vi "Add Or Update Attribute.vi"(8 "error in (no error)":errorcluster, 10 "Atrribute":refnum<class "Attribute.lvclass">, 11 "Object in":refnum<class "Object.lvclass">) -> (0 "error out":errorcluster, 3 "Object out":refnum<class "Object.lvclass">)   [LabVIEW 2019, in "HierDAL Library.lvlib" / "Models.lvlib" / "Object.lvclass"]
uses:
  Object.lvclass
  Attribute Class/Attribute.lvclass
  Object.lvclass/Object.ctl
  Attribute Class/Attribute.lvclass/Attribute.ctl
  d909fb08-bf4f-481c-9526-163c37e898ac.vi
  Attribute Class/Get Key.vi
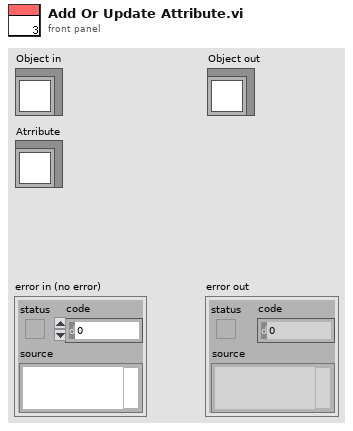
[diagram p1: front panel]
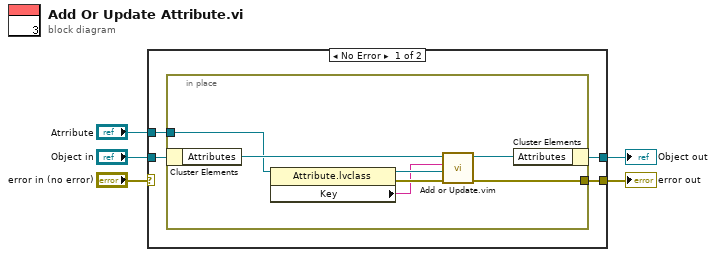
[diagram p0: block diagram]
diagram:
  n1 = case shown="No Error" "error in (no error)" {
    selector: "error in (no error)" -> [_ w18]
    tunnel: [w6 w18] -> w4
    tunnel: [w7 w17] -> w2
    tunnel: "Object in" -> [w9 w17]
    tunnel: "Atrribute" -> [w8 _]
    frame No Error {
      n2 = in-place {
        in-place-border: w8 -> [w14]
        in-place-border: [w10] -> w6
        n3 = in-place-cluster #1(w9) -> ("Attributes"=w16:refnum<data-value>)
        n4 = property class="Attribute.lvclass"(reference=w14) -> (reference out=w12:refnum<class "Attribute.lvclass">, error out=w13:errorcluster, "Key"=w11:string)  [unwired: 1 in]
        n5 = call "Add or Update.vim"("error in (no error)"=w13, "Value"=w12, "Key"=w11, "Map DVR in"=w16) -> ("error out"=w10:errorcluster, "Map DVR out"=w15:refnum<data-value>)  [unwired: 4 in, 2 out]
        n6 = in-place-cluster #1("Attributes"=w15) -> (w7:refnum<class "Object.lvclass">)
      }
    }
    frame Error {
    }
  }
  "error out" <- w4
  "Object out" <- w2
